vi "Init Module.vi"(8 "error in (no error)":errorcluster, 11 "Singleton Module Admin in":refnum<class "Delacor_lib_QMH_Module Admin.lvclass">) -> (0 "error out":errorcluster, 2 "UI Manager Request Events":T1, 3 "Singleton Module Admin out":refnum<class "Delacor_lib_QMH_Module Admin.lvclass">)   [LabVIEW 2020, in "UI Manager.lvlib"]
doc: "Initialize the module by creating Broadcast Events, Request Events, and synchronization rendezvous.\n____\nHAMPEL SOFTWARE ENGINEERING v2.6.0 (2023-12-19 10:54)"
uses:
  UI Manager.lvlib
  <vilib>/Delacor/Delacor QMH/Libraries/Module Admin_class/Delacor_lib_QMH_Module Admin.lvclass
  Request Events--cluster.ctl
  Stop Argument--cluster.ctl
  Show Panel Argument--cluster.ctl
  Hide Panel Argument--cluster.ctl
  Get Module Execution Status Argument--cluster.ctl
  Show Diagram Argument--cluster.ctl
  Set Run-Time Menu Argument--cluster.ctl
  Show HSE-ABOUT Argument--cluster.ctl
  Show PROJECT-ABOUT Argument--cluster.ctl
  Configure Argument--cluster.ctl
  Prepare Argument--cluster.ctl
  Update Status Bar Argument--cluster.ctl
  Trigger System Message Argument--cluster.ctl
  Add Module to Run-Time Menu Argument--cluster.ctl
  Set Modules Argument--cluster.ctl
  Set Modules (Reply Payload)--cluster.ctl
  Register for Module Events Argument--cluster.ctl
  Libraries/hse-libraries/Source/hse-dqmh/Controls/System Message Argument--cluster.ctl
  Libraries/hse-libraries/Source/hse-dqmh/Controls/System Message Source.ctl
  Display another Module UI Argument--cluster.ctl
  Module Display Scenarios.ctl
  Set Run-Time Menu Visibility Argument--cluster.ctl
  Set Window Closeable State Argument--cluster.ctl
  Shutdown Application Argument--cluster.ctl
  Remove Module from Run-Time Menu Argument--cluster.ctl
  Set CLI Arguments Argument--cluster.ctl
  Set CLI Arguments (Reply Payload)--cluster.ctl
  Get CLI Arguments Argument--cluster.ctl
  Get CLI Arguments (Reply Payload)--cluster.ctl
  External Login Argument--cluster.ctl
  Get User Level Argument--cluster.ctl
  Get User Level (Reply Payload)--cluster.ctl
  Libraries/hse-libraries/Source/hse-dqmh/hse-dqmh.lvlib
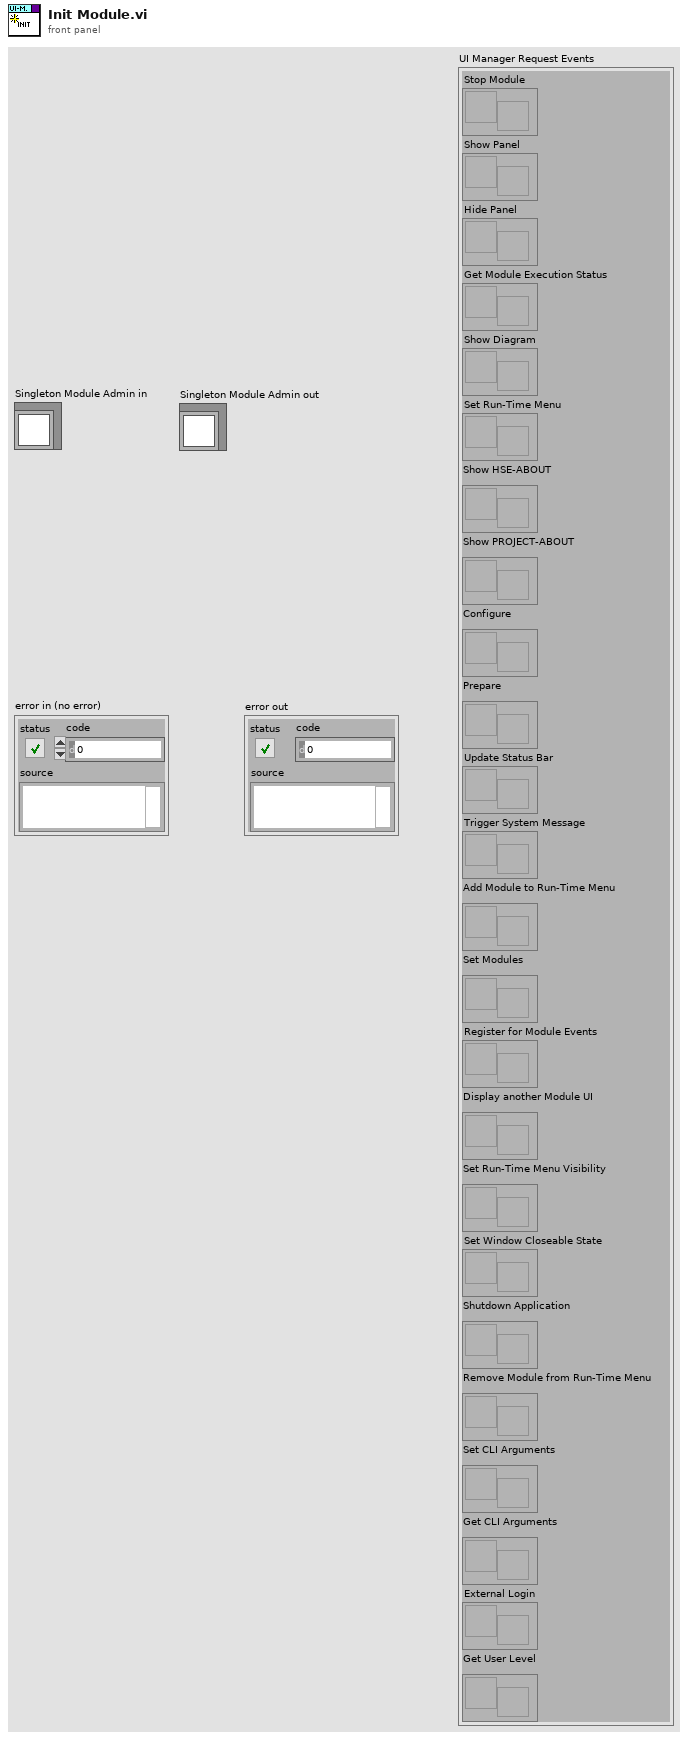
[diagram p1: front panel]
types:
  T1 = typedef "UI Manager.lvlib/Request Events--cluster.ctl" = cluster{"Stop Module":refnum<user-event>, "Show Panel":refnum<user-event>, "Hide Panel":refnum<user-event>, "Get Module Execution Status":refnum<user-event>, "Show Diagram":refnum<user-event>, "Set Run-Time Menu":refnum<user-event>, "Show HSE-ABOUT":refnum<user-event>, "Show PROJECT-ABOUT":refnum<user-event>, "Configure":refnum<user-event>, "Prepare":refnum<user-event>, "Update Status Bar":refnum<user-event>, "Trigger System Message":refnum<user-event>, "Add Module to Run-Time Menu":refnum<user-event>, "Set Modules":refnum<user-event>, "Register for Module Events":refnum<user-event>, "Display another Module UI":refnum<user-event>, "Set Run-Time Menu Visibility":refnum<user-event>, "Set Window Closeable State":refnum<user-event>, "Shutdown Application":refnum<user-event>, "Remove Module from Run-Time Menu":refnum<user-event>, "Set CLI Arguments":refnum<user-event>, "Get CLI Arguments":refnum<user-event>, "External Login":refnum<user-event>, "Get User Level":refnum<user-event>}
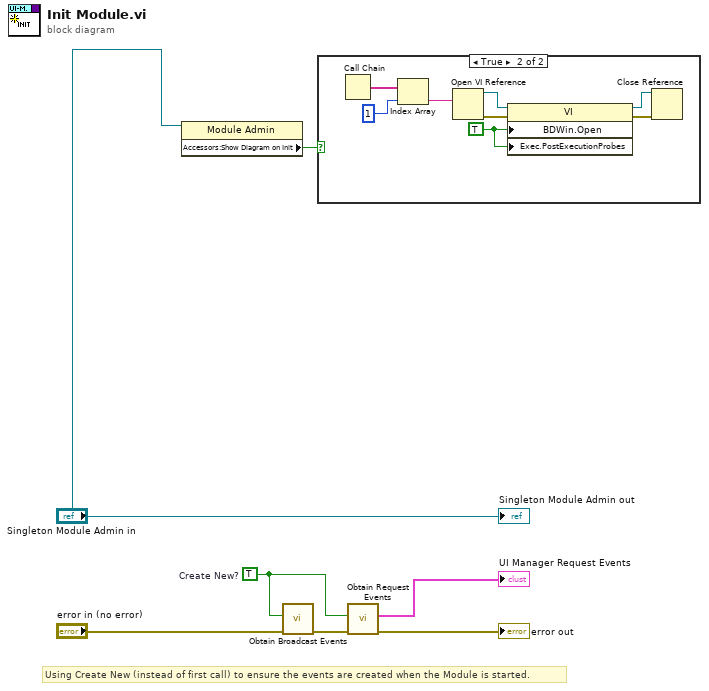
[diagram p0: block diagram]
diagram:
  w4 = TRUE  # Create New?
  # "Using Create New (instead of first call) to ensure the events are created when the Module is started."
  n1 = property class="Module Admin"(reference="Singleton Module Admin in") -> ("Accessors:Show Diagram on Init"=w1:bool)  [unwired: 1 in, 2 out]
  n2 = call "Obtain Broadcast Events.vi"("error in (no error)"="error in (no error)", "Create New?"=w4) -> ("error out"=w7:errorcluster)  [unwired: 8 in, 1 out]
  n3 = case shown="True" w1 {
    frame False {
    }
    frame True {
      w11 = TRUE ("Block Diagram Window:Open")
      n4 = Call Chain() -> (call chain=w15:string[])
      n5 = Index Array(array=w15, index=1) -> (element=w8:string)
      n6 = Open VI Reference(vi path=w8) -> (vi reference=w12:refnum<vi>, error out=w13:errorcluster)  [unwired: 5 in]
      n7 = property class="VI"(reference=w12, error in=w13, "BDWin.Open"=w11, "Exec.PostExecutionProbes"=w11) -> (reference out=w9:refnum<vi>, error out=w10:errorcluster)
      n8 = Close Reference(reference=w9, error in (no error)=w10) -> ()  [unwired: 1 out]
    }
  }
  n9 = call "Obtain Request Events.vi"("error in (no error)"=w7, "Create New?"=w4) -> ("error out"=→"error out":errorcluster, "UI Manager Request Events"=→"UI Manager Request Events":T1)  [unwired: 8 in]
  "Singleton Module Admin out" <- "Singleton Module Admin in"
